vi "Analog Input Voltages.vi"(8 "error in (no error)":errorcluster, 10 "Analog Input Voltages":waveform(dbl)[](array[waveform]), 11 "Top Level in":refnum<class "Top Level.lvclass">) -> (0 "error out":errorcluster, 3 "Top Level out":refnum<class "Top Level.lvclass">)   [LabVIEW 2021, in "Top Level.lvlib" / "Top Level.lvclass"]
uses:
  Top Level.lvclass
  Top Level.lvclass/Top Level.ctl
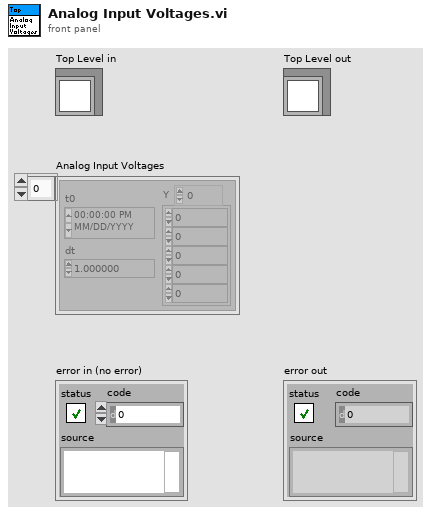
[diagram p1: front panel]
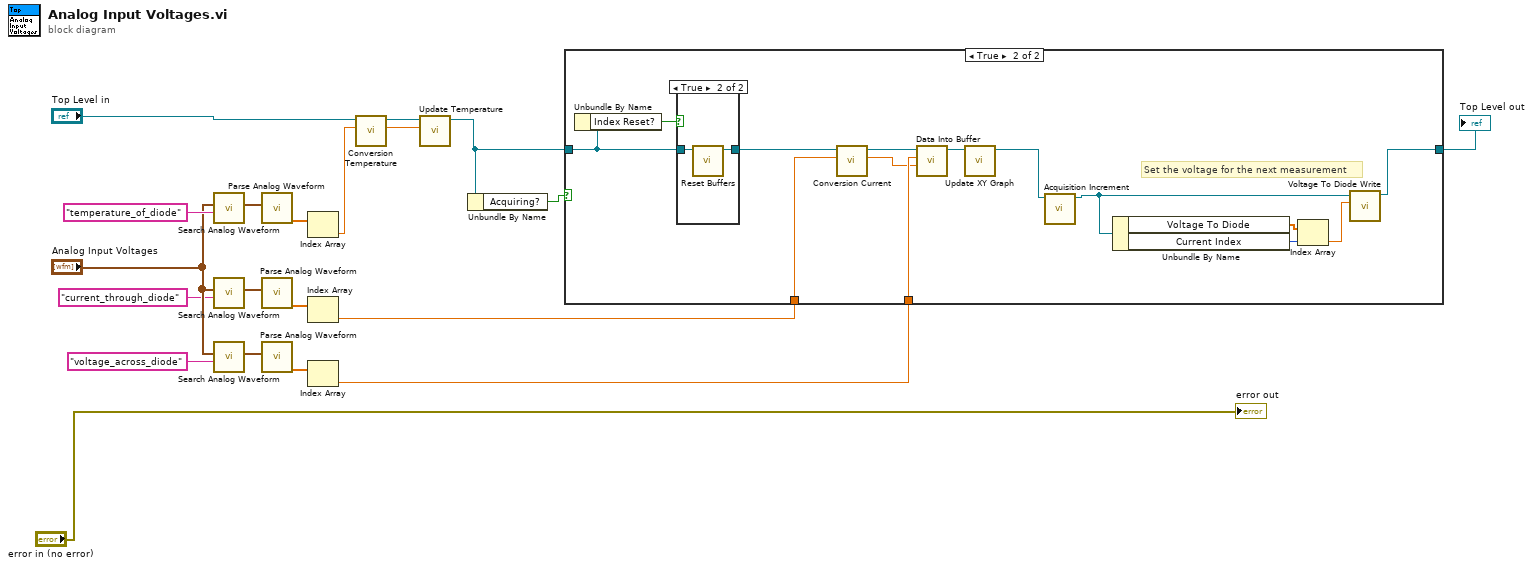
[diagram p0: block diagram]
diagram:
  n1 = call <vilib>:"Search Analog Waveform.vi"("NI_ChannelName"="temperature_of_diode", "Waveforms"="Analog Input Voltages") -> ("Waveform"=w18:waveform(dbl))  [unwired: 8 in, 1 out]
  n2 = call <vilib>:"Search Analog Waveform.vi"("NI_ChannelName"="current_through_diode", "Waveforms"="Analog Input Voltages") -> ("Waveform"=w19:waveform(dbl))  [unwired: 8 in, 1 out]
  n3 = call <vilib>:"Search Analog Waveform.vi"("NI_ChannelName"="voltage_across_diode", "Waveforms"="Analog Input Voltages") -> ("Waveform"=w20:waveform(dbl))  [unwired: 8 in, 1 out]
  n4 = call <vilib>:"Parse Analog Waveform.vi"("Waveform"=w18) -> ("Y"=w16:dbl[])  [unwired: 7 in, 3 out]
  n5 = call <vilib>:"Parse Analog Waveform.vi"("Waveform"=w19) -> ("Y"=w15:dbl[])  [unwired: 7 in, 3 out]
  n6 = call <vilib>:"Parse Analog Waveform.vi"("Waveform"=w20) -> ("Y"=w14:dbl[])  [unwired: 7 in, 3 out]
  n7 = Index Array(array=w16) -> (element=w9:dbl)  [unwired: 1 in]
  n8 = Index Array(array=w15) -> (element=w8:dbl)  [unwired: 1 in]
  n9 = Index Array(array=w14) -> (element=w5:dbl)  [unwired: 1 in]
  n10 = call "Conversion Temperature.vi"("Input"=w9, "Top Level in"="Top Level in") -> ("Output"=w6:dbl, "Top Level out"=w7:refnum<class "Top Level.lvclass">)  [unwired: 7 in, 1 out]
  n11 = call "Update Temperature.vi"("Temperature"=w6, "Top Level in"=w7) -> ("Top Level out"=w4:refnum<class "Top Level.lvclass">)  [unwired: 8 in, 1 out]
  n12 = Unbundle By Name(w4) -> ("Acquiring?"=w3:bool)
  n13 = case shown="True" w3 {
    tunnel: [w21 w28] -> w2
    tunnel: w5 -> [_ w35]
    tunnel: w4 -> [w21 w27]
    tunnel: w8 -> [_ w23]
    frame False {
    }
    frame True {
      # "Set the voltage for the next measurement"
      n14 = Unbundle By Name(w27) -> ("Index Reset?"=w26:bool)
      n15 = case shown="True" w26 {
        tunnel: w27 -> [w36 w38]
        tunnel: [w36 w37] -> w25
        frame False {
        }
        frame True {
          n16 = call "Reset Buffers.vi"("Top Level in"=w38) -> ("Top Level out"=w37:refnum<class "Top Level.lvclass">)  [unwired: 9 in, 1 out]
        }
      }
      n17 = call "Conversion Current.vi"("Input"=w23, "Top Level in"=w25) -> ("Output"=w22:dbl, "Top Level out"=w24:refnum<class "Top Level.lvclass">)  [unwired: 7 in, 1 out]
      n18 = call "Data Into Buffer.vi"("Current Through Diode"=w22, "Voltage Across Diode"=w35, "Top Level in"=w24) -> ("Top Level out"=w34:refnum<class "Top Level.lvclass">)  [unwired: 7 in, 1 out]
      n19 = call "Update XY Graph.vi"("Top Level in"=w34) -> ("Top Level out"=w29:refnum<class "Top Level.lvclass">)  [unwired: 9 in, 1 out]
      n20 = call "Acquisition Increment.vi"("Top Level in"=w29) -> ("Top Level out"=w30:refnum<class "Top Level.lvclass">)  [unwired: 9 in, 1 out]
      n21 = Unbundle By Name(w30) -> ("Voltage To Diode"=w33:dbl[], "Current Index"=w32:i32)
      n22 = Index Array(array=w33, index=w32) -> (element=w31:dbl)
      n23 = call "Voltage To Diode Write.vi"("Voltage"=w31, "Top Level in"=w30) -> ("Top Level out"=w28:refnum<class "Top Level.lvclass">)  [unwired: 8 in, 1 out]
    }
  }
  "Top Level out" <- w2
  "error out" <- "error in (no error)"
